vi "SetAngleHeadingTester.vi"() -> ()   [LabVIEW 2011]
uses:
  <vilib>/robotics/Controls/Compass Indicator/Compass Indicator.xctl
panel:
  out "Compass Heading Out":dbl(xcontrol)
  out "Compass Input Indicatior":dbl(xcontrol)
  out "Relative Heading Out (rad)":dbl
  out "Relative Heading Out (deg)":dbl
  in  "Desired Heading (deg)":dbl(knob) scale=-360.0..360.0
  in  "Curent Heading (deg)":dbl(knob) scale=-360.0..360.0
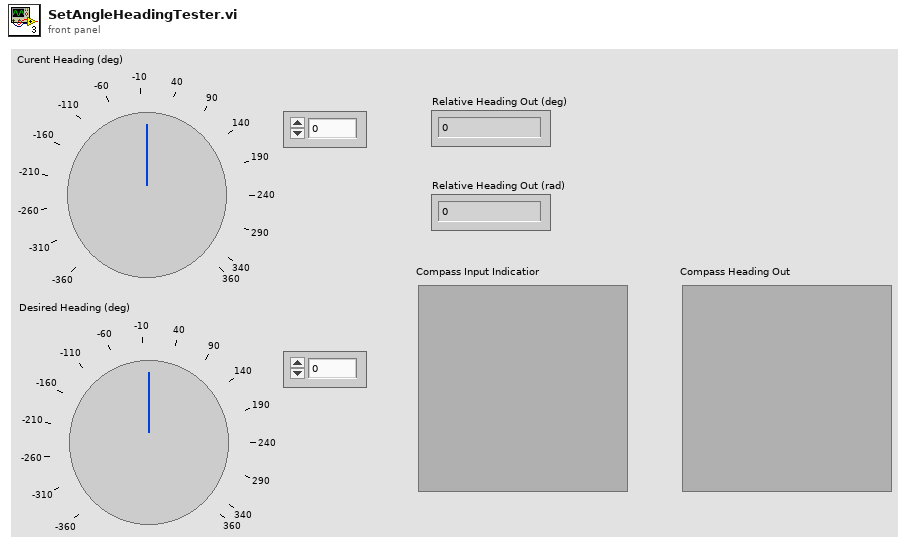
[diagram p1: front panel]
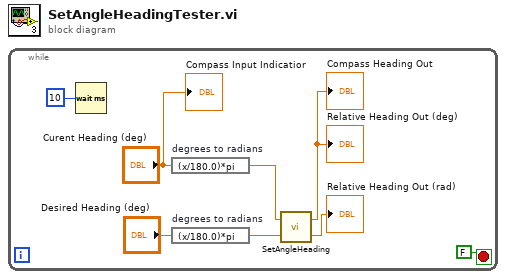
[diagram p0: block diagram]
diagram:
  n1 = while {
    stop <- FALSE stop-if-true
    n2 = Wait (ms)(milliseconds to wait=u32 10) -> ()  [unwired: 1 out]
    n3 = expression code="(x/180.0)*pi" "degrees to radians"("Curent Heading (deg)") -> (w8:dbl)
    n4 = expression code="(x/180.0)*pi" "degrees to radians"("Desired Heading (deg)") -> (w7:dbl)
    n5 = call "SetAngleHeading.vi"("Desired Heading (rad)"=w7, "Current Heading (rad)"=w8) -> ("Relative Angle Out (rad)"=→"Relative Heading Out (rad)":dbl, "Relative Angle Out (deg)"=→"Relative Heading Out (deg)" →"Compass Heading Out":dbl)
    "Compass Input Indicatior" <- "Curent Heading (deg)"
  }
